vi "Index Array.vi"(10 "Backlog":i32, 11 "ApplicationNumberOfWeldChannels":i32) -> (3 "Index":i32)   [LabVIEW 2019, in "SupportVIs.lvlib"]
uses:
  SupportVIs.lvlib
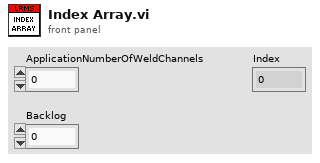
[diagram p1: front panel]
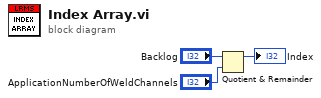
[diagram p0: block diagram]
diagram:
  n1 = Quotient & Remainder(x="Backlog", y="ApplicationNumberOfWeldChannels") -> (x-y*floor(x/y)=→"Index":i32)  [unwired: 1 out]
